vi "Gran plot.vi"(0 "sample":cluster{"Vo":dbl, "Na":dbl, "Measuring":bool} {"Na" format="%.4f"; "Vo" format="%.3f"}, 5 "current":T1 {"Va" format="%.2f"; "temperature" format="%.2f"; "channel 2" format="%.2f"; "channel 1" format="%.2f"}, 9 "sensitivity":dbl=1.0 min=1.0 max=3.0 step=0.01 format="%.2f", 11 "min points":u8) -> (4 "Gran plot":T2={"F1"=[], "Va"=[], "Ve"=0.5, "Alkalinity"=0.5, "r"=0.5, "graph"=[], "Measuring"=FALSE} {"graph"."F1" format="%.2f"; "graph"."Va" format="%.2f"; "r" format="%.6f"; "Alkalinity" format="%.6f"; "Ve" format="%.6f"; "Va" format="%.5f"; "F1" format="%.7f"})   [LabVIEW 2010]
panel:
  # "Normality of titrant"
  # "eq/L"
  # "mL"
  # "Volume of sample"
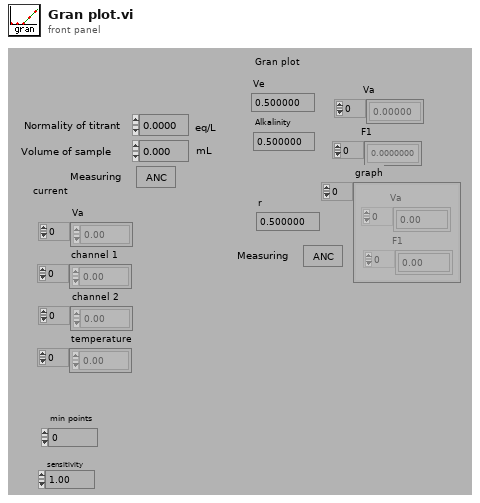
[diagram p1: front panel]
types:
  T1 = cluster{"channel 1":dbl[], "channel 2":dbl[], "temperature":dbl[], "Va":dbl[]}
  T2 = cluster{"F1":dbl[], "Va":dbl[], "Ve":dbl, "Alkalinity":dbl, "r":dbl, "graph":cluster{"Va":dbl[], "F1":dbl[]}[], "Measuring":bool}
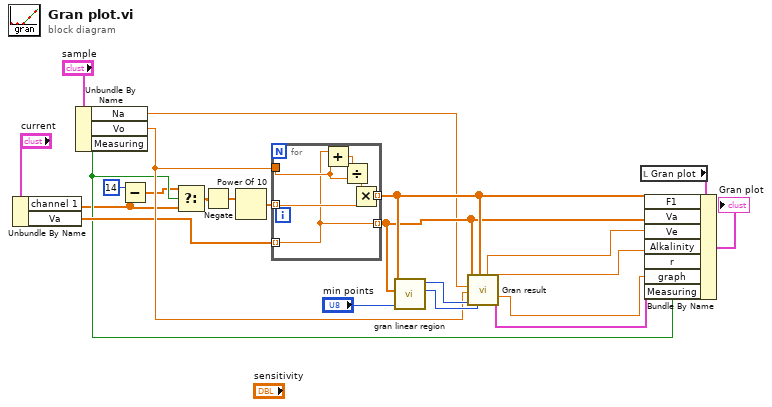
[diagram p0: block diagram]
diagram:
  n1 = Unbundle By Name("current") -> ("channel 1"=w3:dbl[], "Va"=w7:dbl[])
  n2 = Unbundle By Name("sample") -> ("Na"=w9:dbl, "Vo"=w10:dbl, "Measuring"=w6:bool)
  n3 = Subtract(x=14, y=w3) -> (x-y=w1:dbl[])
  n4 = Select(t=w1, s=w6, f=w3) -> (s? t:f=w5:dbl[])
  n5 = Negate(x=w5) -> (-x=w4:dbl[])
  n6 = Power Of 10(x=w4) -> (10^x=w23:dbl[])
  n7 = for {
    tunnel: w23 -> [w28] mode=indexing
    tunnel: [w25] -> w16 mode=indexing
    tunnel: w7 -> [w24] mode=indexing
    tunnel: w10 -> [w26]
    tunnel: [w24] -> w15 mode=indexing
    n8 = Add(x=w24, y=w26) -> (x+y=w29:dbl)
    n9 = Divide(x=w29, y=w26) -> (x/y=w27:dbl)
    n10 = Multiply(x=w27, y=w28) -> (x*y=w25:dbl)
  }
  n11 = call "gran linear region.vi"("min points"="min points", "Va"=w15, "F1"=w16) -> ("first i"=w13:u8, "length"=w14:u8)  [unwired: 7 in]
  n12 = call "Gran result.vi"("first i"=w13, "F1"=w16, "length"=w14, "Vo"=w10, "Nt"=w9, "Vt"=w15) -> ("graph"=w17:cluster{"Vt":dbl[], "F1":dbl[]}[], "r"=w20:dbl, "ANC"=w21:dbl, "Ve"=w22:dbl)  [unwired: 1 in, 1 out]
  n13 = local read "Gran plot"() -> (w19:T2)
  n14 = Bundle By Name(cluster=w19, "F1"=w16, "Va"=w15, "Ve"=w22, "Alkalinity"=w21, "r"=w20, "graph"=w17, "Measuring"=w6) -> (→"Gran plot":T2)
